vi "niScope Configure Horizontal Timing.vi"(0 "instrument handle":refnum<k15>, 1 "number of records":i32=1, 2 "enforce realtime":bool=TRUE, 5 "min sample rate":dbl=20000000.0 format="%^.2e", 9 "reference position":dbl=50.0 format="%.1f", 11 "error in":errorcluster, 12 "min record length":i32=1000) -> (4 "instrument handle out":refnum<k15>, 15 "error out":errorcluster)   [LabVIEW 2020]
doc: "Configures the common properties of the horizontal subsystem for a single record or multirecord acquisition, such as minimum sample rate and acquisition size."
uses:
  niScope_32.dll
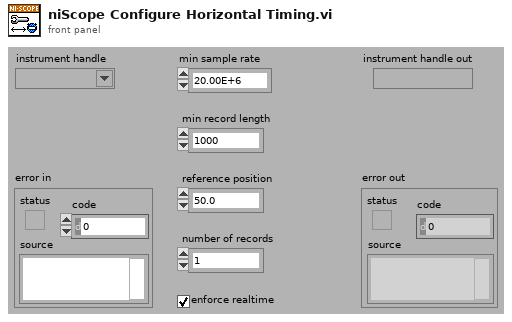
[diagram p1: front panel]
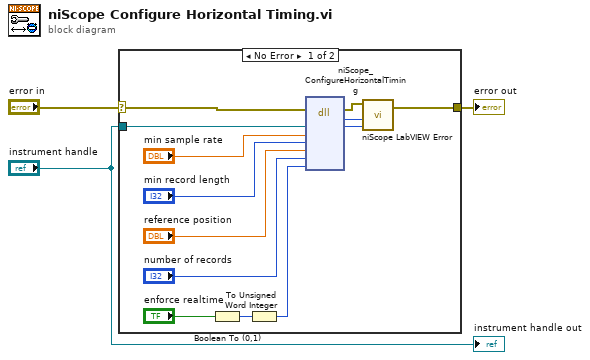
[diagram p0: block diagram]
diagram:
  n1 = case shown="No Error" "error in" {
    selector: "error in" -> [w5 w17]
    tunnel: [w9 w17] -> w3
    tunnel: "instrument handle" -> [w16 _]
    frame No Error {
      n2 = Boolean To (0,1)(Boolean="enforce realtime") -> (0, 1=w7:i16)
      n3 = To Unsigned Word Integer(number=w7) -> (unsigned 16bit integer=w6:u16)
      n4 = dll-call lib="niScope_*.*" fn="niScope_ConfigureHorizontalTiming"(error in=w5, "instrument handle"=w16, "minSampleRate"="min sample rate", "minNumPts"="min record length", "refPosition"="reference position", "numRecords"="number of records", "enforceRealtime"=w6) -> (error out=w4:errorcluster, "status"=w11:i32, "instrument handle"=w10:u32)  [unwired: 7 in, 1 out]
      n5 = call "niScope LabVIEW Error.vi"("instrument handle"=w10, "niScope error code (0)"=w11, "error in (no error)"=w4) -> ("error out"=w9:errorcluster)  [unwired: 2 in]
    }
    frame Error {
    }
  }
  "error out" <- w3
  "instrument handle out" <- "instrument handle"
